vi "EminemStateMachine.vi"(5 "EminemCommand":bool[](array[boolean]), 7 "EminemCancel":bool, 8 "LowerShoot_At_Speed":bool, 9 "UpperShoot_At_Speed":bool) -> (0 "Box states":T1=enum."13-AmpDone", 1 "AmpAndFeed-MotorDmd":dbl, 2 "LowerShooter-RPM_Dmd":dbl, 3 "UpperShooterAndAmp-RPM_Dmd":dbl)   [LabVIEW 2023]
doc: "Process Intake State Machine"
uses:
  EminemStatesEnum.ctl
  <vilib>/Rock Robotics/WPI/ThirdParty/JAS_Junk/TrajLib/Trajectory_Library.lvlib
  EminemGlobals.vi
panel:
  # "Click here to set min"
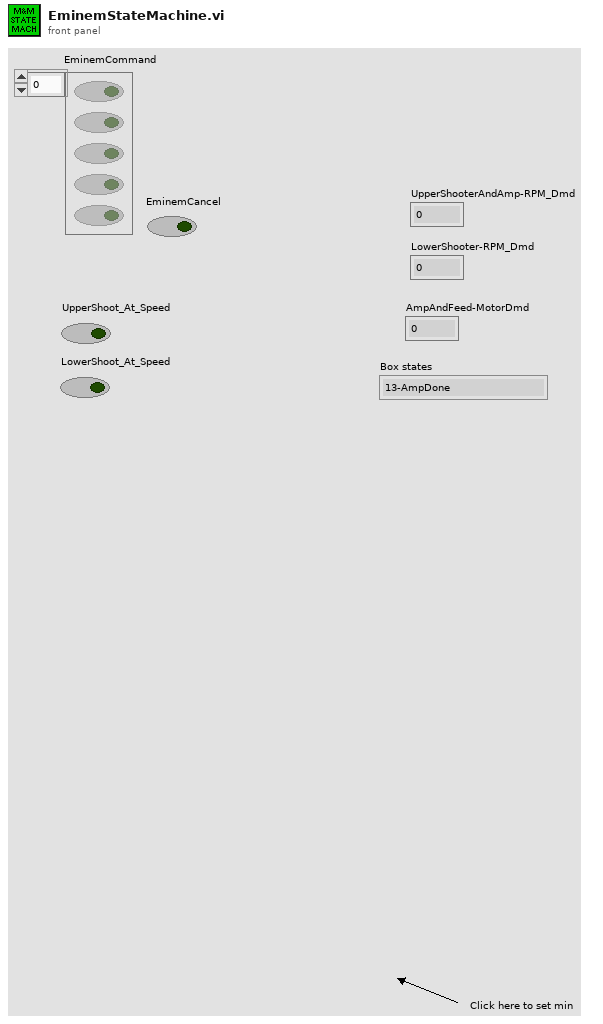
[diagram p1: front panel]
types:
  T1 = typedef "EminemStatesEnum.ctl" = enum16{"0-Init", "1-WaitForCmd", "2-Cancel", "3-ShootStart", "4-ShootRev", "5-RevUpStart", "6-ShootStartFeed&Timer", "7-ShootTimerOrSensorDone", "8-ShootDone", "9-AmpStart", "10-AmpUpToSpd?", "11-AmpStartFeed&Timer", "12-AmpTimerOrSensorDone", "13-AmpDone", "14-RevUpGetCmd"}
  T2 = typedef "Trajectory_Library.lvlib/TIMER.ctl" = cluster{"StartTime":dbl, "Accumulated TIme":dbl, "Running":bool, "semaphore":T3}
  T3 = typedef "Semaphore RefNum" = refnum<k1>
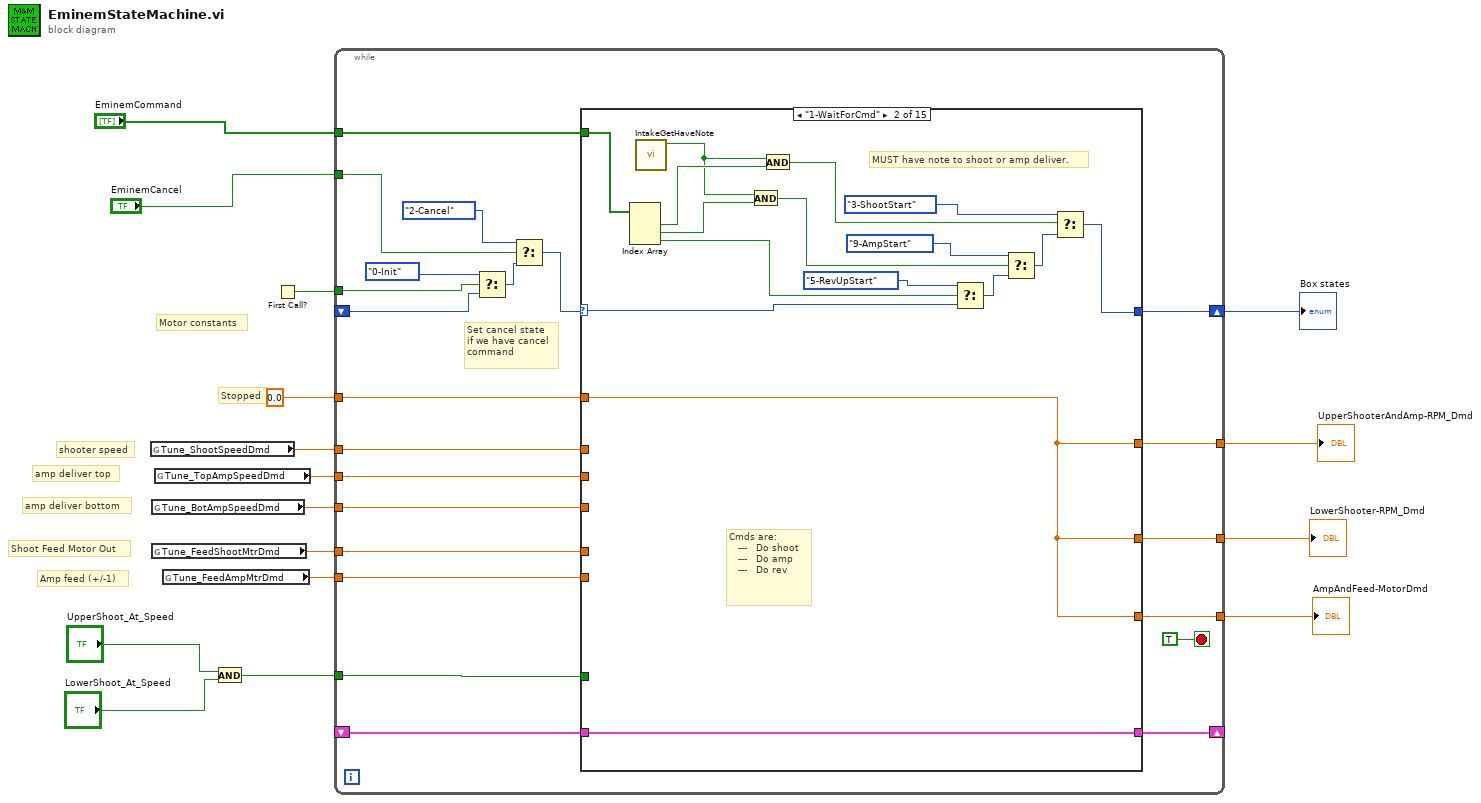
[diagram p0: block diagram]
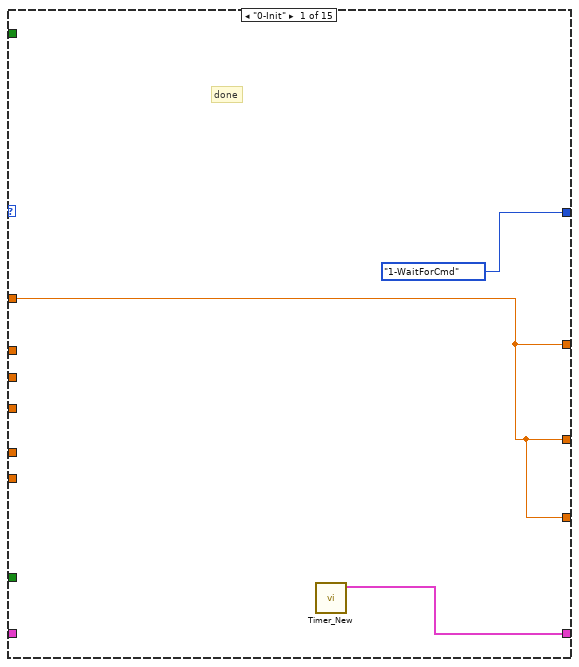
[diagram p2: hidden frame]
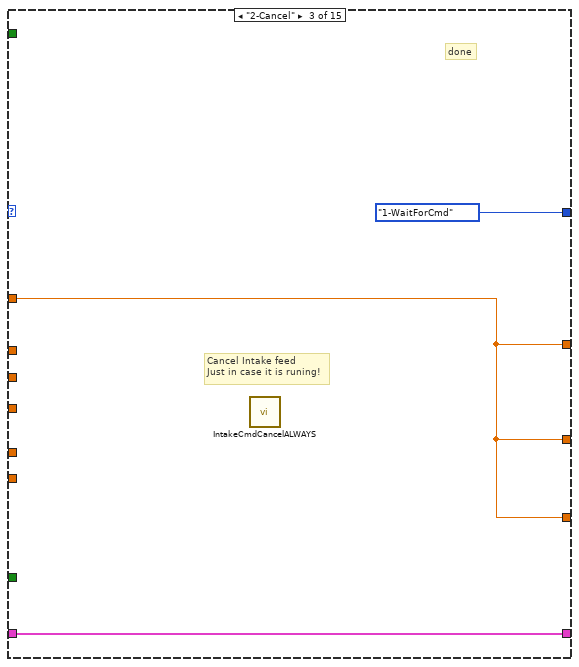
[diagram p3: hidden frame]
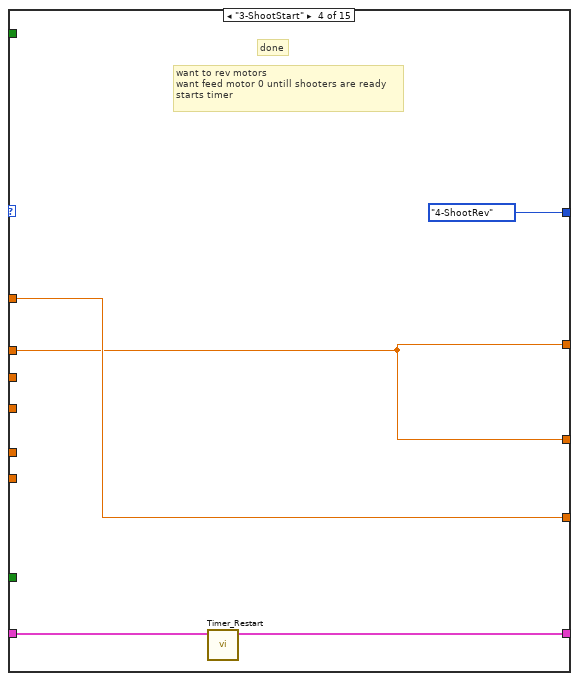
[diagram p4: hidden frame]
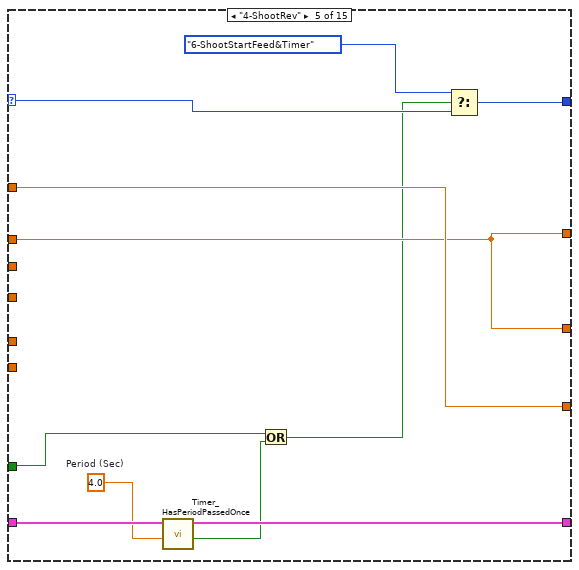
[diagram p5: hidden frame]
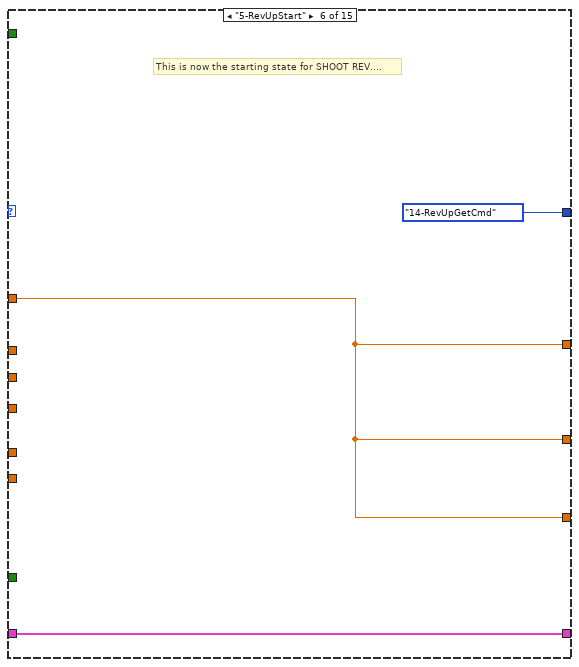
[diagram p6: hidden frame]
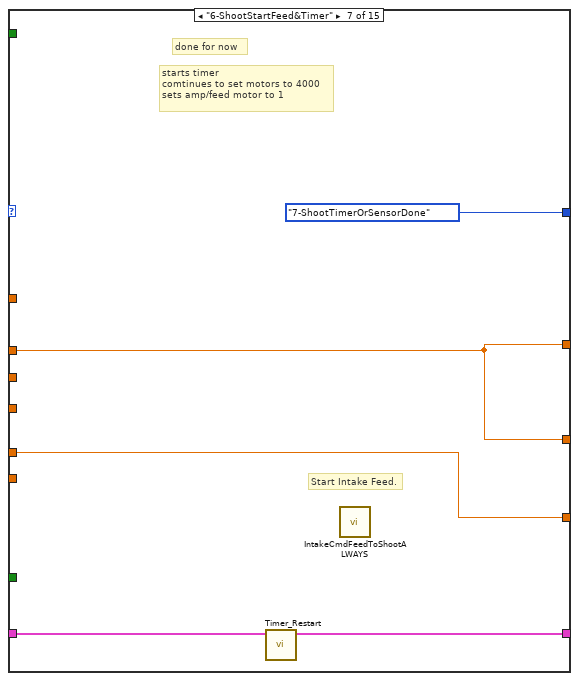
[diagram p7: hidden frame]
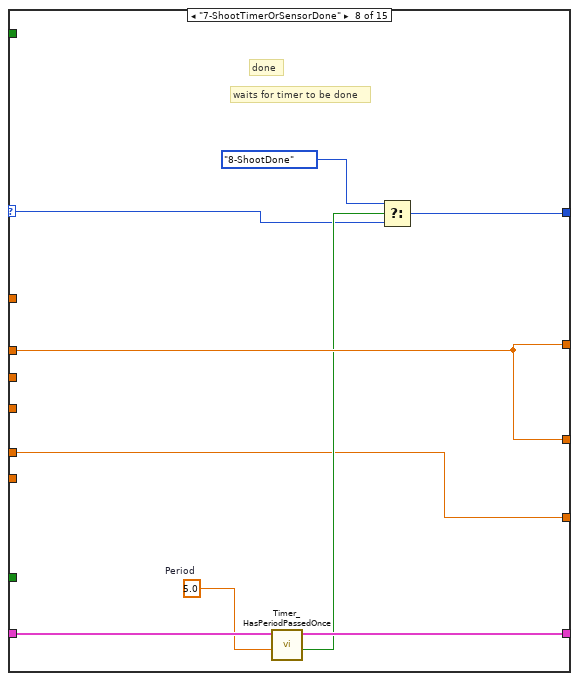
[diagram p8: hidden frame]
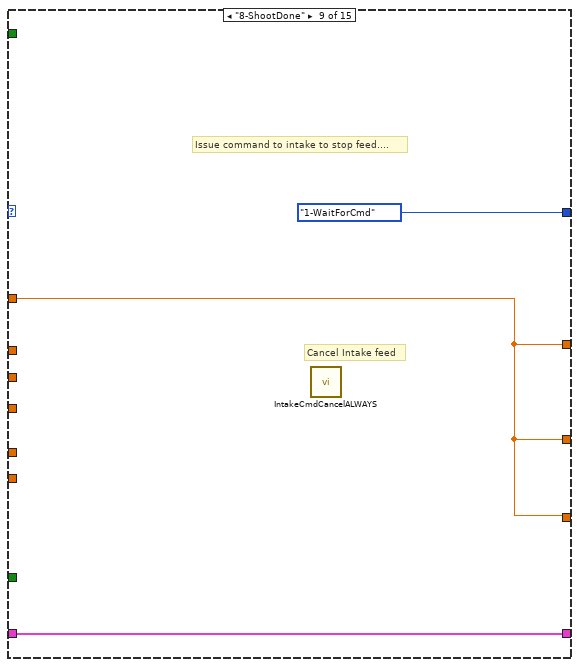
[diagram p9: hidden frame]
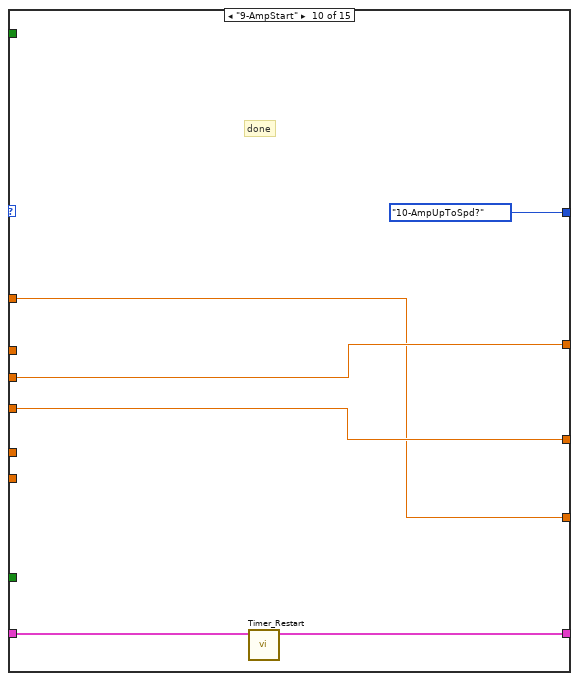
[diagram p10: hidden frame]
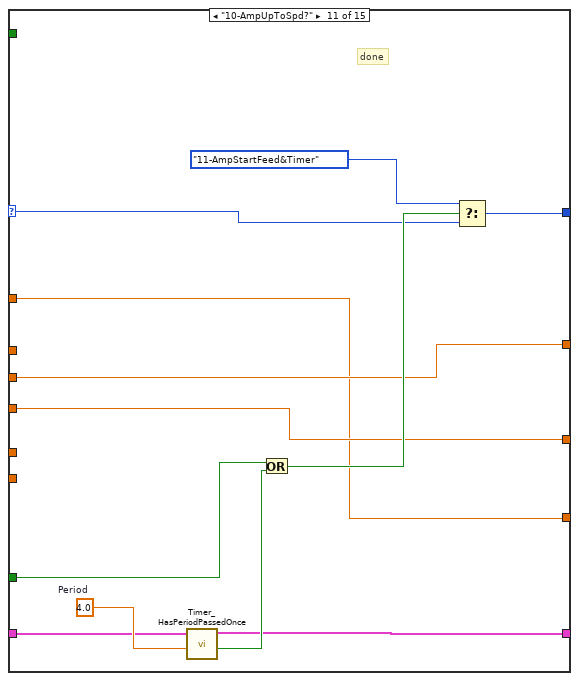
[diagram p11: hidden frame]
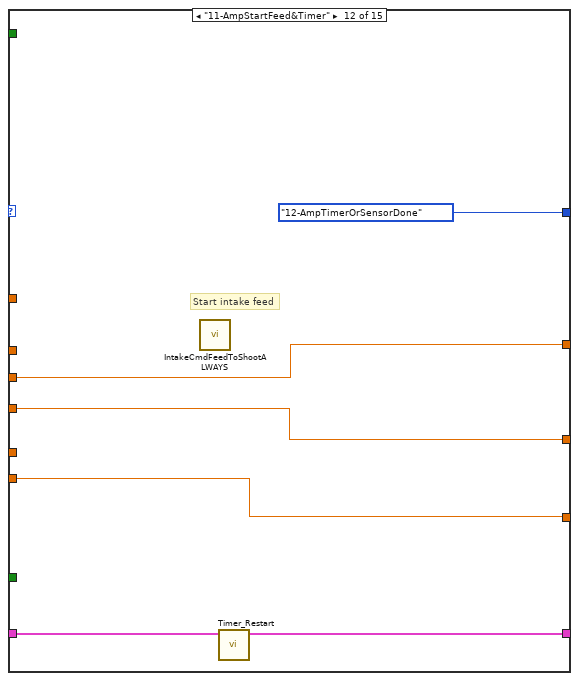
[diagram p12: hidden frame]
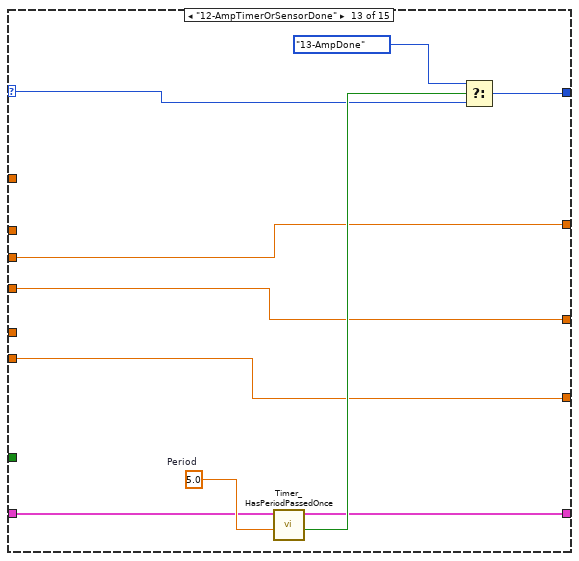
[diagram p13: hidden frame]
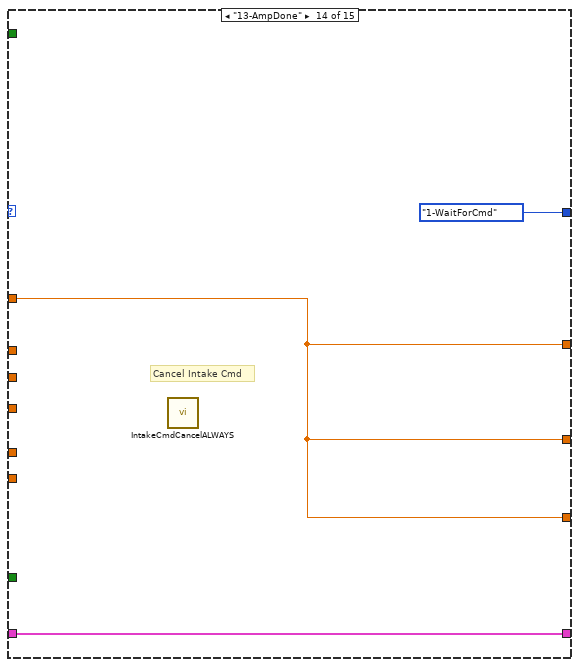
[diagram p14: hidden frame]
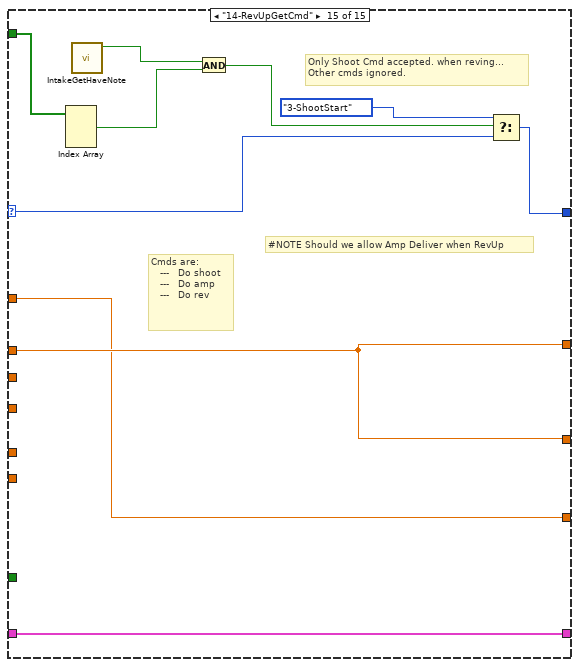
[diagram p15: hidden frame]
diagram:
  # "amp deliver bottom"
  # "amp deliver top"
  # "Amp feed (+/-1)"
  # "shooter speed"
  # "Shoot Feed Motor Out"
  # "Stopped"
  # "Motor constants"
  n1 = global read "EminemGlobals.vi" "Tune_ShootSpeedDmd"() -> (w1:dbl)
  n2 = global read "EminemGlobals.vi" "Tune_BotAmpSpeedDmd"() -> (w3:dbl)
  n3 = global read "EminemGlobals.vi" "Tune_FeedShootMtrDmd"() -> (w4:dbl)
  n4 = global read "EminemGlobals.vi" "Tune_TopAmpSpeedDmd"() -> (w2:dbl)
  n5 = global read "EminemGlobals.vi" "Tune_FeedAmpMtrDmd"() -> (w5:dbl)
  n6 = And(x="UpperShoot_At_Speed", y="LowerShoot_At_Speed") -> (x .and. y?=w6:bool)
  n7 = First Call?() -> (First Call?: T/F=w13:bool)
  n8 = while {
    tunnel: "EminemCommand" -> [w38]
    tunnel: [w37] -> w15
    tunnel: "EminemCancel" -> [w17]
    shift-right: [w27] -> w9
    shift-left: _ -> [w33]
    tunnel: w13 -> [w34]
    tunnel: w4 -> [w32]
    tunnel: 0.0 -> [w31]
    tunnel: [w29] -> w11
    tunnel: [w28] -> w10
    tunnel: w1 -> [w26]
    shift-right: [w25] -> _
    shift-left: _ -> [w24]
    tunnel: w6 -> [w23]
    tunnel: w5 -> [w22]
    tunnel: w2 -> [w21]
    tunnel: w3 -> [w20]
    stop <- TRUE stop-if-true
    # "Set cancel state\nif we have cancel\ncommand"
    n9 = Select(t=EminemStatesEnum."0-Init" ("Box states"), s=w34, f=w33) -> (s? t:f=w35:T1)
    n10 = Select(t=EminemStatesEnum."2-Cancel" ("Box states"), s=w17, f=w35) -> (s? t:f=w18:T1)
    n11 = case shown="\"1-WaitForCmd\"" w18 {
      selector: w18 -> [_ w50 _ _ w72 _ _ w87 _ _ w106 _ w127 _ w138]
      tunnel: [w41 w57 w60 w64 w75 w79 w82 w93 w96 w102 w105 w119 w126 w131 w136] -> w37
      tunnel: w38 -> [_ w51 _ _ _ _ _ _ _ _ _ _ _ _ w140]
      tunnel: w32 -> [_ _ _ _ _ _ w80 w85 _ _ _ _ _ _ _]
      tunnel: w31 -> [w41 w57 w60 w65 w76 w79 _ _ w96 w100 w103 _ _ w131 w135]
      tunnel: [w41 w57 w60 w64 w75 w79 w82 w93 w96 w101 w104 w118 w125 w131 w136] -> w29
      tunnel: [w41 w57 w60 w65 w76 w79 w80 w85 w96 w100 w103 w115 w121 w131 w135] -> w28
      tunnel: [EminemStatesEnum."1-WaitForCmd" ("Box states") w49 EminemStatesEnum."1-WaitForCmd" ("MNM States") EminemStatesEnum."4-ShootRev" ("Box states") w74 EminemStatesEnum."14-RevUpGetCmd" ("Box states") EminemStatesEnum."7-ShootTimerOrSensorDone" ("Box states") w86 EminemStatesEnum."1-WaitForCmd" ("Box states") EminemStatesEnum."10-AmpUpToSpd?" ("Box states") w109 EminemStatesEnum."12-AmpTimerOrSensorDone" ("Box states") w122 EminemStatesEnum."1-WaitForCmd" ("Box states") w137] -> w27
      tunnel: w26 -> [_ _ _ w64 w75 _ w82 w93 _ _ _ _ _ _ w136]
      tunnel: [w39 w48 w58 w63 w70 w78 w83 w91 w94 w99 w110 w116 w124 w132 w134] -> w25
      tunnel: w24 -> [_ w48 w58 w62 w71 w78 w84 w92 w94 w98 w111 w117 w123 w132 w134]
      tunnel: w23 -> [_ _ _ _ w68 _ _ _ _ _ w108 _ _ _ _]
      tunnel: w22 -> [_ _ _ _ _ _ _ _ _ _ _ w115 w121 _ _]
      tunnel: w21 -> [_ _ _ _ _ _ _ _ _ w102 w105 w119 w126 _ _]
      tunnel: w20 -> [_ _ _ _ _ _ _ _ _ w101 w104 w118 w125 _ _]
      frame "0-Init" {
        # "done"
        n12 = call <vilib>:"Timer_New.vi"() -> ("TIMER"=w39:T2)  [unwired: 11 in]
      }
      frame "1-WaitForCmd" {
        # "MUST have note to shoot or amp deliver."
        # "Cmds are:\n   ---   Do shoot\n   ---   Do amp\n   ---   Do rev"
        n13 = Index Array(array=w51) -> (element #1=w45:bool, element #2=w43:bool, element #3=w53:bool)  [unwired: 3 in]
        n14 = call "IntakeGetHaveNote.vi"() -> ("IntakeHaveNote"=w44:bool)  [unwired: 11 in]
        n15 = And(x=w44, y=w43) -> (x .and. y?=w42:bool)
        n16 = And(x=w44, y=w45) -> (x .and. y?=w46:bool)
        n17 = Select(t=EminemStatesEnum."5-RevUpStart" ("Box states"), s=w53, f=w50) -> (s? t:f=w56:T1)
        n18 = Select(t=EminemStatesEnum."9-AmpStart" ("Box states"), s=w42, f=w56) -> (s? t:f=w55:T1)
        n19 = Select(t=EminemStatesEnum."3-ShootStart" ("Box states"), s=w46, f=w55) -> (s? t:f=w49:T1)
      }
      frame "2-Cancel" {
        # "Cancel Intake feed\nJust in case it is runing!"
        # "done"
        n20 = call "IntakeCmdCancelALWAYS.vi"() -> ()  [unwired: 12 in]
      }
      frame "3-ShootStart" {
        # "done"
        # "want to rev motors\nwant feed motor 0 untill shooters are ready\nstarts timer"
        n21 = call <vilib>:"Timer_Restart.vi"("in Timer"=w62) -> ("out Timer"=w63:T2)  [unwired: 10 in]
      }
      frame "4-ShootRev" {
        w69 = 4.0  # Period (Sec)
        n22 = call <vilib>:"Timer_HasPeriodPassedOnce.vi"("Period"=w69, "in Timer"=w71) -> ("Expired"=w67:bool, "out Timer"=w70:T2)  [unwired: 7 in, 1 out]
        n23 = Or(x=w68, y=w67) -> (x .or. y?=w66:bool)
        n24 = Select(t=EminemStatesEnum."6-ShootStartFeed&Timer" ("Box states"), s=w66, f=w72) -> (s? t:f=w74:T1)
      }
      frame "5-RevUpStart" {
        # "This is now the starting state for SHOOT REV...."
      }
      frame "6-ShootStartFeed&Timer" {
        # "Start Intake Feed."
        # "done for now"
        # "starts timer\ncomtinues to set motors to 4000\nsets amp/feed motor to 1"
        n25 = call <vilib>:"Timer_Restart.vi"("in Timer"=w84) -> ("out Timer"=w83:T2)  [unwired: 10 in]
        n26 = call "IntakeCmdFeedToShootALWAYS.vi"() -> ()  [unwired: 12 in]
      }
      frame "7-ShootTimerOrSensorDone" {
        w90 = 5.0  # Period
        # "done"
        # "waits for timer to be done"
        n27 = call <vilib>:"Timer_HasPeriodPassedOnce.vi"("Period"=w90, "in Timer"=w92) -> ("Expired"=w89:bool, "out Timer"=w91:T2)  [unwired: 7 in, 1 out]
        n28 = Select(t=EminemStatesEnum."8-ShootDone" ("Box states"), s=w89, f=w87) -> (s? t:f=w86:T1)
      }
      frame "8-ShootDone" {
        # "Cancel Intake feed"
        # "Issue command to intake to stop feed...."
        n29 = call "IntakeCmdCancelALWAYS.vi"() -> ()  [unwired: 12 in]
      }
      frame "9-AmpStart" {
        # "done"
        n30 = call <vilib>:"Timer_Restart.vi"("in Timer"=w98) -> ("out Timer"=w99:T2)  [unwired: 10 in]
      }
      frame "10-AmpUpToSpd?" {
        w113 = 4.0  # Period
        # "done"
        n31 = call <vilib>:"Timer_HasPeriodPassedOnce.vi"("Period"=w113, "in Timer"=w111) -> ("Expired"=w112:bool, "out Timer"=w110:T2)  [unwired: 7 in, 1 out]
        n32 = Or(x=w108, y=w112) -> (x .or. y?=w107:bool)
        n33 = Select(t=EminemStatesEnum."11-AmpStartFeed&Timer" ("Box states"), s=w107, f=w106) -> (s? t:f=w109:T1)
      }
      frame "11-AmpStartFeed&Timer" {
        # "Start intake feed"
        n34 = call "IntakeCmdFeedToShootALWAYS.vi"() -> ()  [unwired: 12 in]
        n35 = call <vilib>:"Timer_Restart.vi"("in Timer"=w117) -> ("out Timer"=w116:T2)  [unwired: 10 in]
      }
      frame "12-AmpTimerOrSensorDone" {
        w130 = 5.0  # Period
        n36 = call <vilib>:"Timer_HasPeriodPassedOnce.vi"("Period"=w130, "in Timer"=w123) -> ("Expired"=w129:bool, "out Timer"=w124:T2)  [unwired: 7 in, 1 out]
        n37 = Select(t=EminemStatesEnum."13-AmpDone" ("Box states"), s=w129, f=w127) -> (s? t:f=w122:T1)
      }
      frame "13-AmpDone" {
        # "Cancel Intake Cmd"
        n38 = call "IntakeCmdCancelALWAYS.vi"() -> ()  [unwired: 12 in]
      }
      frame "14-RevUpGetCmd" {
        # "#NOTE Should we allow Amp Deliver when RevUp"
        # "Only Shoot Cmd accepted. when reving...\nOther cmds ignored."
        # "Cmds are:\n   ---   Do shoot\n   ---   Do amp\n   ---   Do rev"
        n39 = Index Array(array=w140) -> (element #1=w139:bool)  [unwired: 3 in, 2 out]
        n40 = call "IntakeGetHaveNote.vi"() -> ("IntakeHaveNote"=w141:bool)  [unwired: 11 in]
        n41 = And(x=w141, y=w139) -> (x .and. y?=w142:bool)
        n42 = Select(t=EminemStatesEnum."3-ShootStart" ("Box states"), s=w142, f=w138) -> (s? t:f=w137:T1)
      }
    }
  }
  "UpperShooterAndAmp-RPM_Dmd" <- w15
  "AmpAndFeed-MotorDmd" <- w10
  "LowerShooter-RPM_Dmd" <- w11
  "Box states" <- w9
